vi "Gantry.vi"(0 "COMPORT":string="COM5", 5 "error in (no error)":errorcluster, 6 "Use manual(t)":bool, 7 "Antenna Select":u16(ring)=1 items=["HOME", "TX1", "TX2", "TX3", "TX4", "TX5", "TX6", "TX7", "TX8", "TX9", "TX10", "TX11", "TX12", "RX8", "RX7", "RX6", "RX5", "RX4", "RX3", "RX2", "RX1"], 8 "EnableDriver(t)":bool=TRUE, 9 "z ref":dbl=21.0 format="%#_6f", 10 "Write(reads antenna co-ords when off)":bool=TRUE, 11 "z":dbl=21.0 format="%#_6f", 13 "Zunits":u16(ring) items=["Inches", "cm"]) -> (19 "error out":errorcluster)   [LabVIEW 2018]
uses:
  Initialize References/Sequence Globals.vi
  <vilib>/Utility/file.llb/Read Delimited Spreadsheet (DBL).vi
panel:
  in  "Close Serial":bool
  in  "y":dbl format="%#_13g"
  in  "x":dbl
  out "y":dbl=638961.0
  out "x":dbl=156330.0
  out "time":dbl=4.024529500005883
  out "begin":dbl=83230.42149349999 format="%_19f"
  out "return value":string[](array[string])=["638961.0", "156330.0"]
  out "List":dbl[][](array[numeric])=[[0.0, 0.0, 0.0, 247141.0, 0.0, 52711.0, 103619.0], [156330.0, 638961.0, 0.0, 247141.0, 0.0, 0.0, 103619.0], [193621.0, 638961.0, 0.0, 284432.0, 0.0, 0.0, 140910.0], [230912.0, 638961.0, 0.0, 321723.0, 0.0, 0.0, 178201.0], [268203.0, 638961.0, 0.0, 359014.0, 0.0, 0.0, 215492.0], [305494.0, 638961.0, 0.0, 396305.0, 0.0, 0.0, 252783.0], [342785.0, 638961.0, 0.0, 433596.0, 0.0, 0.0, 290074.0], [380076.0, 638961.0, 0.0, 470887.0, 0.0, 0.0, 327365.0], [417367.0, 638961.0, 0.0, 508178.0, 0.0, 0.0, 364656.0], [454658.0, 638961.0, 0.0, 545469.0, 0.0, 0.0, 401947.0], [491949.0, 638961.0, 0.0, 582760.0, 0.0, 0.0, 439238.0], [529240.0, 638961.0, 0.0, 620051.0, 0.0, 0.0, 476529.0], [566531.0, 638961.0, 0.0, 657342.0, 0.0, 0.0, 513820.0], [556452.0, 873796.0, 0.0, 647263.0, 0.0, 0.0, 503741.0], [500440.0, 873796.0, 0.0, 591251.0, 0.0, 0.0, 447729.0], [444428.0, 873796.0, 0.0, 535239.0, 0.0, 0.0, 391717.0], [388416.0, 873796.0, 0.0, 479227.0, 0.0, 0.0, 335705.0], [332404.0, 873796.0, 0.0, 423215.0, 0.0, 0.0, 279693.0], [276392.0, 873796.0, 0.0, 367203.0, 0.0, 0.0, 223681.0], [220380.0, 873796.0, 0.0, 311191.0, 0.0, 0.0, 167669.0], [164368.0, 873796.0, 0.0, 255179.0, 0.0, 0.0, 111657.0], [0.0, 0.0, 0.0, 0.0, 0.0, 0.0, 0.0], [0.0, 0.0, 0.0, 0.0, 0.0, 0.0, 0.0], [0.0, 0.0, 0.0, 0.0, 0.0, 0.0, 0.0]]
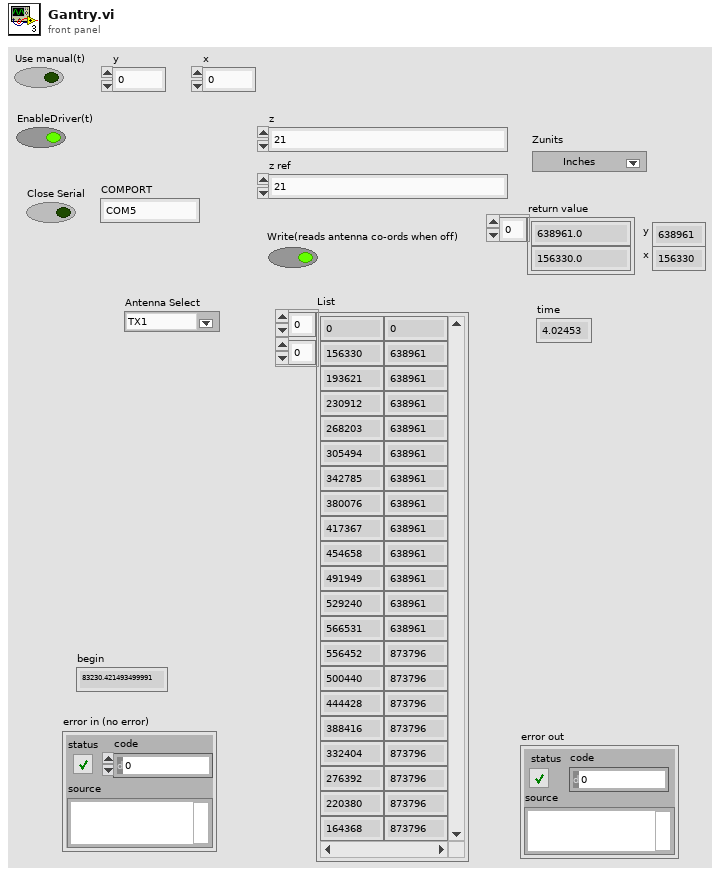
[diagram p1: front panel]
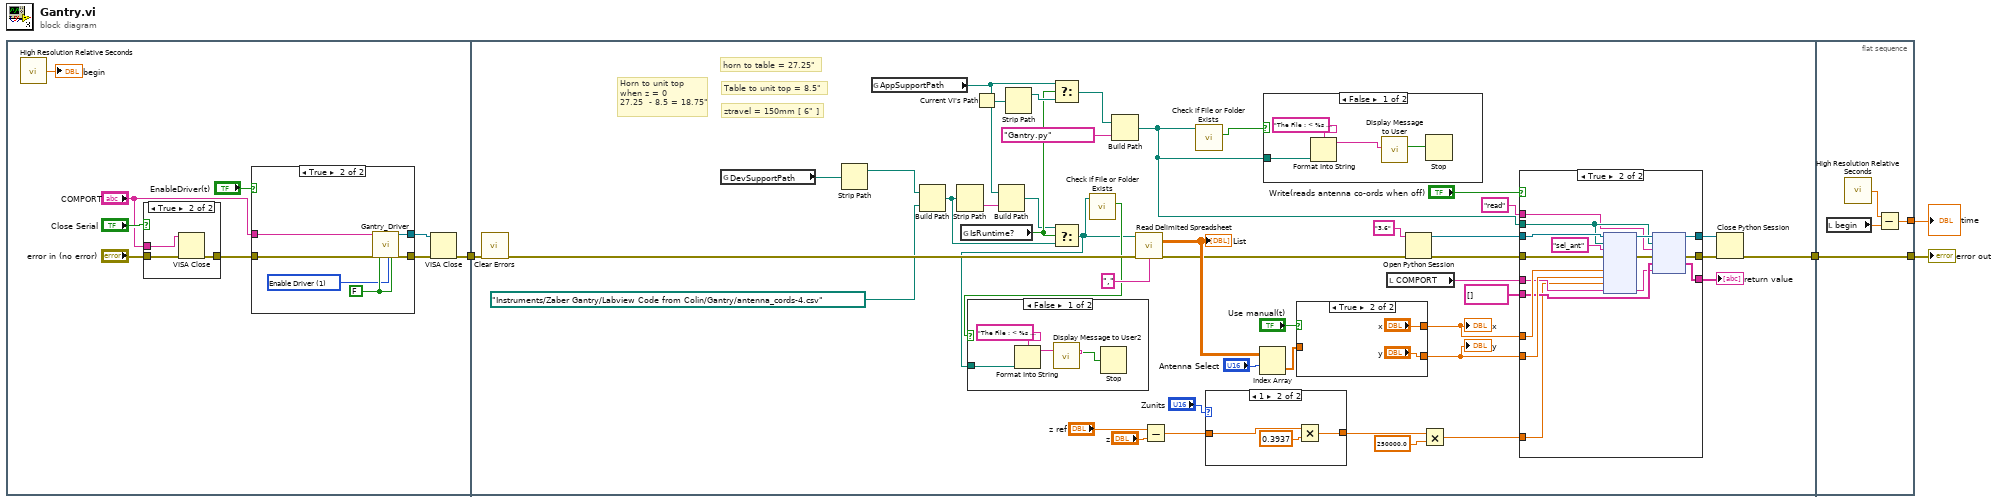
[diagram p0: block diagram]
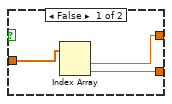
[diagram p7: hidden frame]
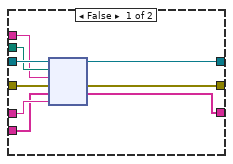
[diagram p8: hidden frame]
diagram:
  n1 = flat-sequence {
    tunnel: [w7] -> w1
    tunnel: [w69] -> w3
    tunnel: w1 -> [w41]
    tunnel: [w114] -> w4
    tunnel: w3 -> [w112]
    tunnel: [w112] -> w2
    frame #0 {
      n2 = call <vilib>:"High Resolution Relative Seconds.vi"() -> ("relative seconds"=→"begin":dbl)
      n3 = case shown="True" "Close Serial" {
        tunnel: "error in (no error)" -> [w14 w17]
        tunnel: [w14 w16] -> w10
        tunnel: "COMPORT" -> [_ w15]
        frame False {
        }
        frame True {
          n4 = VISA Close(VISA resource name=w15, error in (no error)=w17) -> (error out=w16:errorcluster)
        }
      }
      n5 = case shown="True" "EnableDriver(t)" {
        tunnel: "COMPORT" -> [w18 w25]
        tunnel: w10 -> [w19 w24]
        tunnel: [w19 w21] -> w8
        tunnel: [w18 w20] -> w6
        frame False {
        }
        frame True {
          w22 = u16 1 items=["Disable Driver", "Enable Driver", "Read Driver Status"] ("Driver-Func")
          w23 = FALSE ("Close Serial")
          n6 = call "Gantry_Driver.vi"("VISA resource name"=w25, "error in (no error)"=w24, "Open Serial"=w23, "Driver-Func"=w22, "Close Serial"=w23) -> ("VISA resource name out"=w20:refnum<visa-resource-name>, "error out"=w21:errorcluster)  [unwired: 11 in, 2 out]
        }
      }
      n7 = VISA Close(VISA resource name=w6, error in (no error)=w8) -> (error out=w7:errorcluster)
    }
    frame #1 {
      # "Horn to unit top \nwhen z = 0\n27.25  - 8.5 = 18.75\""
      # "ztravel = 150mm [ 6\" ]"
      # "Table to unit top = 8.5\""
      # "horn to table = 27.25\""
      n8 = call <vilib>:"Clear Errors.vi"("error in (no error)"=w41) -> ("error out"=w42:errorcluster)  [unwired: 5 in, 1 out]
      n9 = global read "Sequence Globals.vi" "DevSupportPath"() -> (w33:path)
      n10 = Strip Path(path=w33) -> (stripped path=w31:path)  [unwired: 1 out]
      n11 = global read "Sequence Globals.vi" "AppSupportPath"() -> (w35:path)
      n12 = Build Path(base path=w31, name or relative path=path "Instruments/Zaber Gantry/Labview Code from Colin/Gantry/antenna_cords-4.csv" ("file path (dialog if empty)")) -> (appended path=w32:path)
      n13 = Strip Path(path=w32) -> (name=w34:string)  [unwired: 1 out]
      n14 = global read "Sequence Globals.vi" "IsRuntime?"() -> (w37:bool)
      n15 = Current VI's Path() -> (path=w59:path)
      n16 = Build Path(base path=w35, name or relative path=w34) -> (appended path=w36:path)
      n17 = Strip Path(path=w59) -> (stripped path=w38:path)  [unwired: 1 out]
      n18 = Select(t=w35, s=w37, f=w38) -> (s? t:f=w39:path)
      n19 = Select(t=w36, s=w37, f=w32) -> (s? t:f=w26:path)
      n20 = call <vilib>:"Check if File or Folder Exists.vi"("path"=w26) -> ("file or folder exists?"=w27:bool)  [unwired: 8 in, 2 out]
      n21 = case shown="False" w27 {
        tunnel: w26 -> [w72 _]
        frame False {
          n22 = Format Into String(format string="The File : < %s > does not exist in this location ", w72) -> (resulting string=w71:string)  [unwired: 2 in, 1 out]
          n23 = call "Display Message to User2"("Message"=w71) -> ("OK"=w70:bool)  [unwired: 9 in, 1 out]
          n24 = Stop(stop? (T)=w70) -> ()
        }
        frame True {
        }
      }
      n25 = Build Path(base path=w39, name or relative path="Gantry.py") -> (appended path=w28:path)
      n26 = call-poly <vilib>:"Read Delimited Spreadsheet.vi"("file path (dialog if empty)"=w26, "error in (no error)"=w42, "delimiter (\\t)"="," ("delimiter (\\t)")) -> ("all rows"=w65:dbl[][], "error out"=w57:errorcluster)  [unwired: 7 in, 4 out]
      "List" <- w65
      n27 = Subtract(x="z ref", y="z") -> (x-y=w45:dbl)
      n28 = call <vilib>:"Check if File or Folder Exists.vi"("path"=w28) -> ("file or folder exists?"=w29:bool)  [unwired: 8 in, 2 out]
      n29 = case shown="1" "Zunits" {
        tunnel: w45 -> [w78 w80]
        tunnel: [w78 w79] -> w46
        frame 0, Default {
        }
        frame 1 {
          n30 = Multiply(x=w80, y=0.3937) -> (x*y=w79:dbl)
        }
      }
      n31 = Index Array(array=w65, index (row)="Antenna Select") -> (element=w63:dbl[])  [unwired: 1 in]
      n32 = case shown="False" w29 {
        tunnel: w28 -> [w76 _]
        frame False {
          n33 = Format Into String(format string="The File : < %s > does not exist in this location ", w76) -> (resulting string=w75:string)  [unwired: 2 in, 1 out]
          n34 = call "Display Message to User"("Message"=w75) -> ("OK"=w74:bool)  [unwired: 9 in, 1 out]
          n35 = Stop(stop? (T)=w74) -> ()
        }
        frame True {
        }
      }
      n36 = case shown="True" "Use manual(t)" {
        tunnel: w63 -> [w84 _]
        tunnel: [w83 "x"] -> w62
        tunnel: [w82 "y"] -> w61
        frame False {
          n37 = Index Array(array=w84) -> (element #1=w83:dbl, element #2=w82:dbl)  [unwired: 2 in]
        }
        frame True {
        }
      }
      "x" <- w62
      "y" <- w61
      n38 = local read "COMPORT"() -> (w40:string)
      n39 = Open Python Session(python version="3.6" ("Python version"), 3:w57) -> (session out=w56:refnum<k35>, error out=w55:errorcluster)  [unwired: 1 in]
      n40 = Multiply(x=w46, y=250000.0) -> (x*y=w48:dbl)
      n41 = case shown="True" "Write(reads antenna co-ords when off)" {
        tunnel: [w93 w98] -> w67
        tunnel: [w94 w97] -> w66
        tunnel: w62 -> [_ w110]
        tunnel: w61 -> [_ w109]
        tunnel: w28 -> [w91 w105]
        tunnel: w56 -> [w92 w108]
        tunnel: w55 -> [w95 w107]
        tunnel: w40 -> [w90 w101]
        tunnel: [w89 w104] -> w53
        tunnel: string[] [] -> [w88 w103]
        tunnel: "read" ("function name") -> [w87 w102]
        tunnel: w48 -> [_ w96]
        frame False {
          n42 = node(w92, w91, w87, w95, w88, w90) -> (w93:refnum<k35>, w94:errorcluster, w89:string[])  [unwired: 1 in, 2 out]
        }
        frame True {
          n43 = node(w108, w105, "sel_ant" ("function name"), w107, w110, w109, w96, w101) -> (w106:refnum<k35>, w99:errorcluster, w100:string)  [unwired: 5 in, 2 out]
          n44 = node(w106, w105, w102, w99, w103, w100) -> (w98:refnum<k35>, w97:errorcluster, w104:string[])  [unwired: 1 in, 2 out]
        }
      }
      "return value" <- w53
      n45 = Close Python Session(session in=w67, error in=w66) -> (11:w69:errorcluster)
    }
    frame #2 {
      n46 = local read "begin"() -> (w113:dbl)
      n47 = call <vilib>:"High Resolution Relative Seconds.vi"() -> ("relative seconds"=w115:dbl)
      n48 = Subtract(x=w115, y=w113) -> (x-y=w114:dbl)
    }
  }
  "time" <- w4
  "error out" <- w2
